vi "PV ActiveLine - AD Converter.vi"(8 "Fehler (Eingang)":errorcluster, 10 "A/D Converter":string(combo)="TAD", 11 "Referenz in":refnum<visa-resource-name>) -> (0 "Cluster (Ausgang)":errorcluster, 1 "Channel 2":dbl format="%.4f", 2 "Channel 1":dbl format="%.4f", 3 "Referenz out":refnum<visa-resource-name>)   [LabVIEW 2013, in "PV ActiveLine.lvlib"]
doc: "ADC Test A/D Converter and TAI - A/D Converter, ID Resistance \n\nTransmit: ADC\nReceive: aa.aaaa,bb.bbbb\n\naa.aaaa = A/D converter channel 1 Measurement signal [0.0000 … 11.0000 V]\nbb.bbbb = A/D converter channel 2 Measurement signal [0.0000 … 11.0000 V]\n\n\nTransmit: TAI\nReceive: a.aa,b.bb\n\na.aa = Identification resistance gauge 1 [kOhm]\nb.bb = Identification resistance gauge 2 [kOhm]"
uses:
  <instrlib>/PV ActiveLine/PV ActiveLine.lvlib
panel:
  # "V"
  # "V"
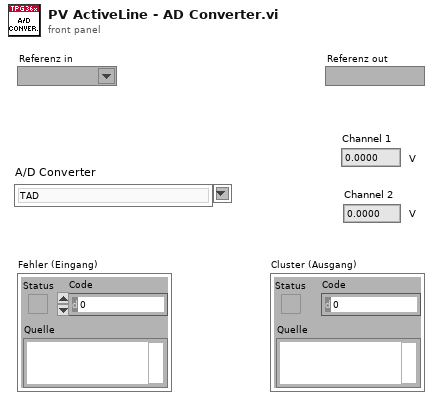
[diagram p1: front panel]
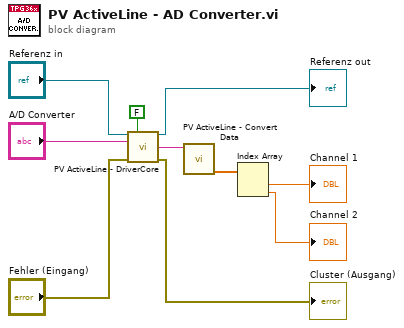
[diagram p0: block diagram]
diagram:
  n1 = call <instrlib>:"PV ActiveLine - DriverCore.vi"("Referenz in"="Referenz in", "Write/Read"=FALSE, "Command"="A/D Converter", "Fehler (Eingang)"="Fehler (Eingang)") -> ("Referenz out"=→"Referenz out":refnum<visa-resource-name>, "String Out"=w4:string, "Cluster (Ausgang)"=→"Cluster (Ausgang)":errorcluster)  [unwired: 9 in]
  n2 = call <instrlib>:"PV ActiveLine - Convert Data.vi"("String in"=w4) -> ("DBL out"=w3:dbl[])  [unwired: 7 in, 3 out]
  n3 = Index Array(array=w3) -> (element #1=→"Channel 1":dbl, element #2=→"Channel 2":dbl)  [unwired: 2 in]
